vi "BK Precision 178XB Run Voltage Transient Output.vi"() -> ()   [LabVIEW 2019]
doc: "This example VI creates a continuous voltage transient between two voltage values with a specified timing between each."
uses:
  BK Precision 178XB Series.lvlib
panel:
  in  "Current Limit (0)":dbl min=0.0 max=6.0 format="%#.2g"
  in  "Maximum Output Voltage (18)":dbl=18.0 min=0.0 max=72.0 step=1.0 format="%#.2g"
  in  "Voltage A (0)":dbl min=0.0 max=72.0 format="%#.2g"
  in  "Voltage B (0)":dbl min=0.0 max=72.0 format="%#.2g"
  in  "Time B (1000)":u16=1000 min=100
  in  "Time A (1000)":u16=1000 min=100
  in  "VISA resource name":refnum<visa-resource-name>
  in  "stop":bool
  # "Instructions:  Input the max. output voltage as the overvoltage protection limit.  Then setup the current limiting value.  Voltage A and Voltage B are the values to create the transient.  Time A corresponds to timing to hold Voltage A before changing to Voltage B.  Time B is the timing to hold Voltage B before changing back to Voltage A."
  # "(c) 2009 B&K PRECISION CORPORATION.  ALL RIGHTS RESERVED."
  # "A"
  # "V"
  # "V"
  # "V"
  # "ms"
  # "ms"
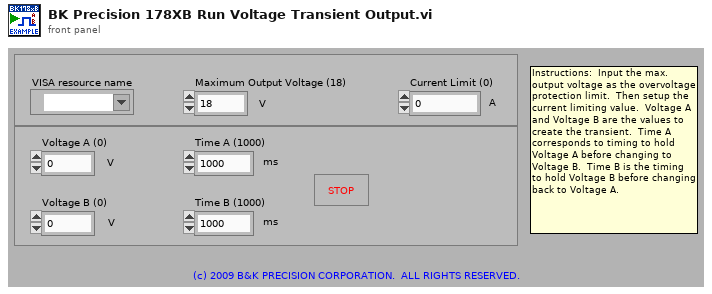
[diagram p1: front panel]
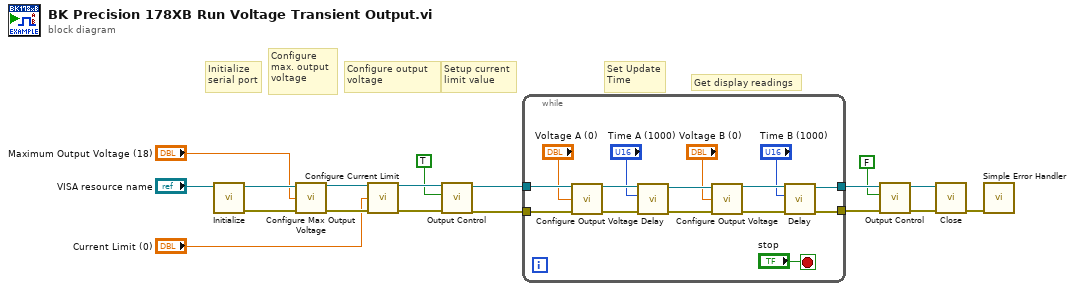
[diagram p0: block diagram]
diagram:
  # "Setup current\nlimit value"
  # "Configure output\nvoltage"
  # "Configure\nmax. output\nvoltage"
  # "Initialize\nserial port"
  # "Get display readings"
  # "Set Update\nTime"
  n1 = call "Initialize.vi"("VISA resource name"="VISA resource name") -> ("error out"=w16:errorcluster, "VISA resource name out"=w17:refnum<visa-resource-name>)  [unwired: 9 in]
  n2 = call "Configure Max Output Voltage.vi"("VISA resource name"=w17, "Maximum Output Voltage (18)"="Maximum Output Voltage (18)", "error in (no error)"=w16) -> ("VISA resource name out"=w3:refnum<visa-resource-name>, "error out"=w2:errorcluster)  [unwired: 11 in]
  n3 = call "Configure Current Limit.vi"("VISA resource name"=w3, "Current Limit (0)"="Current Limit (0)", "error in (no error)"=w2) -> ("VISA resource name out"=w15:refnum<visa-resource-name>, "error out"=w14:errorcluster)  [unwired: 11 in]
  n4 = call "Output Control.vi"("error in (no error)"=w14, "Enable Output Terminals (F: Off)"=TRUE, "VISA resource name"=w15) -> ("error out"=w9:errorcluster, "VISA resource name out"=w10:refnum<visa-resource-name>)  [unwired: 7 in]
  n5 = while {
    tunnel: [w24] -> w7
    tunnel: [w23] -> w8
    tunnel: w10 -> [w32]
    tunnel: w9 -> [w31]
    stop <- "stop" stop-if-true
    n6 = call "Configure Output Voltage.vi"("VISA resource name"=w32, "Output Voltage (0)"="Voltage A (0)", "error in (no error)"=w31) -> ("VISA resource name out"=w30:refnum<visa-resource-name>, "error out"=w29:errorcluster)  [unwired: 11 in]
    n7 = call "Delay.vi"("error in (no error)"=w29, "Delay Value (100)"="Time A (1000)", "VISA resource name"=w30) -> ("error out"=w25:errorcluster, "VISA resource name out"=w26:refnum<visa-resource-name>)  [unwired: 7 in]
    n8 = call "Configure Output Voltage.vi"("VISA resource name"=w26, "Output Voltage (0)"="Voltage B (0)", "error in (no error)"=w25) -> ("VISA resource name out"=w28:refnum<visa-resource-name>, "error out"=w27:errorcluster)  [unwired: 11 in]
    n9 = call "Delay.vi"("error in (no error)"=w27, "Delay Value (100)"="Time B (1000)", "VISA resource name"=w28) -> ("error out"=w23:errorcluster, "VISA resource name out"=w24:refnum<visa-resource-name>)  [unwired: 7 in]
  }
  n10 = call "Output Control.vi"("error in (no error)"=w8, "Enable Output Terminals (F: Off)"=FALSE, "VISA resource name"=w7) -> ("error out"=w5:errorcluster, "VISA resource name out"=w6:refnum<visa-resource-name>)  [unwired: 7 in]
  n11 = call "Close.vi"("error in (no error)"=w5, "VISA resource name"=w6) -> ("error out"=w18:errorcluster)  [unwired: 9 in]
  n12 = call <vilib>:"Simple Error Handler.vi"("error in (no error)"=w18) -> ()  [unwired: 4 in, 5 out]
